vi "Launch Async.vi"(8 "error in (no error)":errorcluster, 11 "VectoService in":refnum<class "VectoInfo.lvclass">) -> (0 "error out":errorcluster, 3 "VectoService out":refnum<class "VectoInfo.lvclass">)   [LabVIEW 2020, in "Vecto.lvlib" / "VectoInfo.lvclass"]
uses:
  VectoInfo.lvclass
  Vecto Info Async.vi
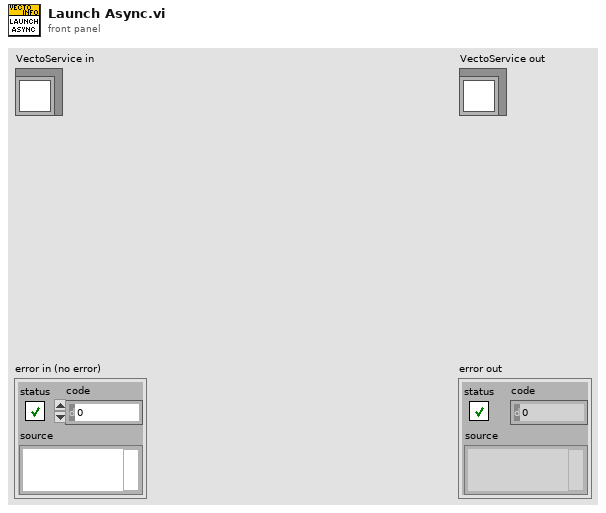
[diagram p1: front panel]
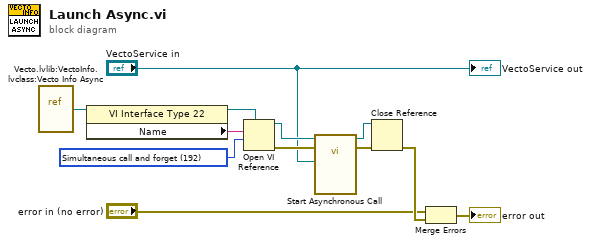
[diagram p0: block diagram]
diagram:
  w7 = 192 items=["Record modifications"=1, "Open templates for editing"=2, "Prompt user to save"=4, "Prepare for reentrant run"=8, "Prompt to find missing subVIs"=16, "Hide loading dialog box"=32, "Enable simultaneous calls"=64, "Prepare to call and forget"=128, "Simultaneous call and forget"=192, "Prepare to call and collect"=256, "Simultaneous call and collect"=320]
  n1 = vi-ref "Vecto.lvlib:VectoInfo.lvclass:Vecto Info Async.vi"() -> (w5:refnum<vi>)
  n2 = property class="VI Interface Type 22"(reference=w5) -> (reference out=w8:refnum<vi>, "Name"=w6:string)  [unwired: 1 in, 1 out]
  n3 = Open VI Reference(type specifier VI Refnum (for type only)=w8, vi path=w6, options=w7) -> (vi reference=w10:refnum<vi>, error out=w9:errorcluster)  [unwired: 3 in]
  n4 = call-by-ref "Start Asynchronous Call"(reference=w10, error in=w9, "VectoService in"="VectoService in") -> (reference out=w12:refnum<vi>, error out=w11:errorcluster)  [unwired: 11 in]
  n5 = Close Reference(reference=w12, error in (no error)=w11) -> (error out=w3:errorcluster)
  n6 = Merge Errors("error in (no error)", w3) -> (→"error out":errorcluster)
  "VectoService out" <- "VectoService in"
